vi "DUPLICATE ITEM.vi"(11 "ITEM DATA IN":T1) -> ()   [LabVIEW 2019]
uses:
  <vilib>/addons/database/Connection.llb/DB Tools Open Connec (String).vi
  <vilib>/regexp/Match Regular Expression.xnode
  <vilib>/addons/database/NI_Database_API.lvlib
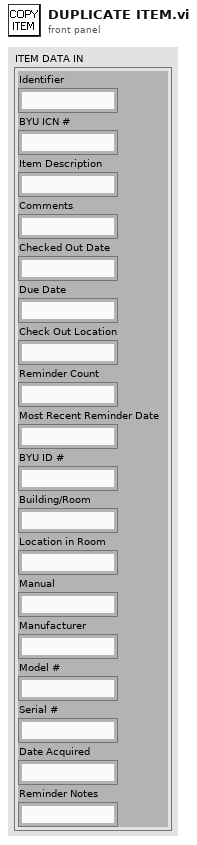
[diagram p1: front panel]
types:
  T1 = cluster{"Identifier":string, "BYU ICN #":string, "Item Description":string, "Comments":string, "Checked Out Date":string, "Due Date":string, "Check Out Location":string, "Reminder Count":string, "Most Recent Reminder Date":string, "BYU ID #":string, "Building/Room":string, "Location in Room":string, "Manual":string, "Manufacturer":string, "Model #":string, "Serial #":string, "Date Acquired":string, "Reminder Notes":string}
  T2 = typedef "NI_Database_API.lvlib/Conn ObjectReference.ctl" = refnum<k1>
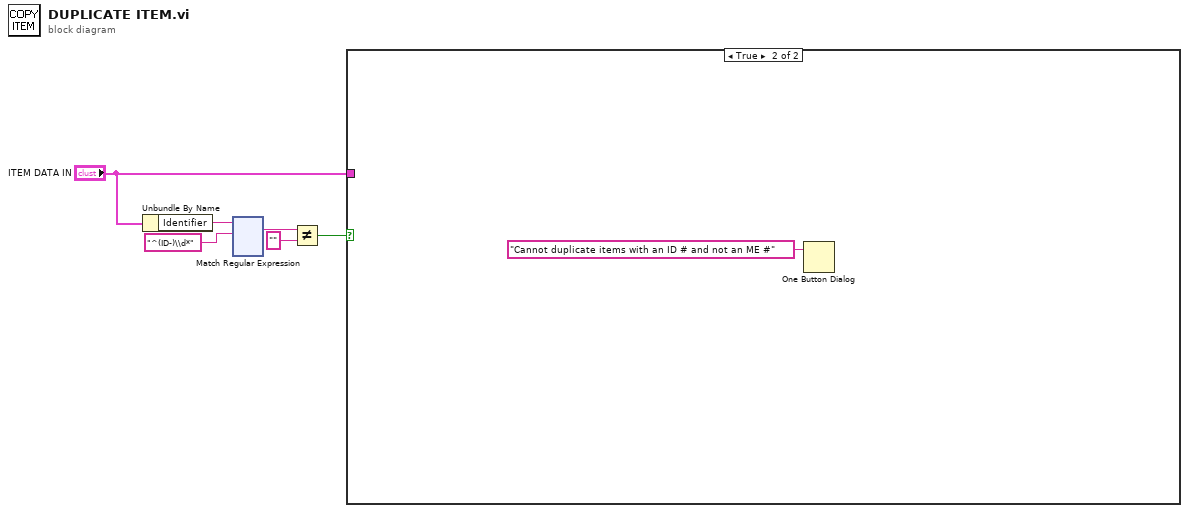
[diagram p0: block diagram]
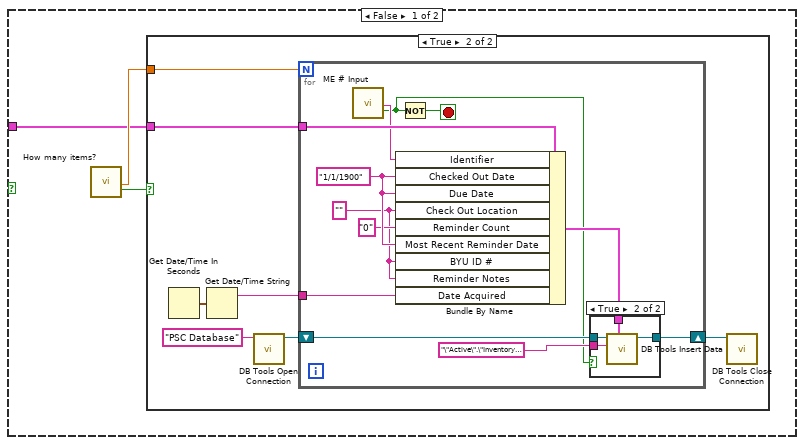
[diagram p2: hidden frame]
diagram:
  n1 = Unbundle By Name("ITEM DATA IN") -> ("Identifier"=w6:string)
  n2 = xnode "Match Regular Expression"("input string"=w6, "regular expression"="^(ID-)\\d*") -> ("whole match"=w4:string)  [unwired: 4 in, 4 out]
  n3 = Not Equal?(x=w4, y="") -> (x != y?=w1:bool)
  n4 = case shown="True" w1 {
    tunnel: "ITEM DATA IN" -> [w7 _]
    frame False {
      n5 = call "How many items?"() -> ("Duplicate Quantity"=w8:dbl, "OK"=w9:bool)  [unwired: 17 in, 1 out]
      n6 = case shown="True" w9 {
        tunnel: w8 -> [_ w14]
        tunnel: w7 -> [_ w13]
        frame False {
        }
        frame True {
          n7 = Get Date/Time In Seconds() -> (seconds since 1Jan1904=w12:timestamp)
          n8 = Get Date/Time String(seconds (now)=w12) -> (date string=w11:string)  [unwired: 2 in, 1 out]
          n9 = call-poly <vilib>:"DB Tools Open Connection.vi"("connection information"="PSC Database") -> ("connection reference"=w15:T2)  [unwired: 7 in, 1 out]
          n10 = for {
            N: w14 -> [_]
            shift-right: [w17] -> w10
            shift-left: w15 -> [w21]
            tunnel: w13 -> [w27]
            tunnel: w11 -> [w24]
            stop <- w28 stop-if-true
            w22 = "" ("Check Out Location")
            w25 = "1/1/1900" ("Checked Out Date")
            n11 = call "ME # Input"() -> ("ME #"=w26:string, "OK"=w18:bool)  [unwired: 17 in, 1 out]
            n12 = Bundle By Name(cluster=w27, "Identifier"=w26, "Checked Out Date"=w25, "Due Date"=w25, "Check Out Location"=w22, "Reminder Count"="0", "Most Recent Reminder Date"=w25, "BYU ID #"=w22, "Reminder Notes"=w22, "Date Acquired"=w24) -> (w19:T1)
            n13 = Not(x=w18) -> (.not. x?=w28:bool)
            n14 = case shown="True" w18 {
              tunnel: w21 -> [w29 w33]
              tunnel: "\"Active\".\"Inventory\"" ("table") -> [_ w32]
              tunnel: w19 -> [_ w31]
              tunnel: [w29 w30] -> w17
              frame False {
              }
              frame True {
                n15 = call <vilib>:"DB Tools Insert Data.vi"("data"=w31, "table"=w32, "connection reference"=w33) -> ("connection reference out"=w30:T2)  [unwired: 7 in, 1 out]
              }
            }
          }
          n16 = call <vilib>:"DB Tools Close Connection.vi"("connection reference"=w10) -> ()  [unwired: 6 in, 1 out]
        }
      }
    }
    frame True {
      n17 = One Button Dialog(message="Cannot duplicate items with an ID # and not an ME #") -> ()  [unwired: 1 in, 1 out]
    }
  }
